vi "op_biti_v5.vi"() -> ()   [LabVIEW 2009]
panel:
  out "Boolean 2":bool=TRUE
  in  "Boolean":bool=TRUE
  out "Array 2":bool[](array[boolean])=[FALSE, FALSE, FALSE, FALSE, FALSE, FALSE, FALSE, TRUE]
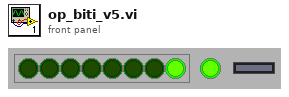
[diagram p1: front panel]
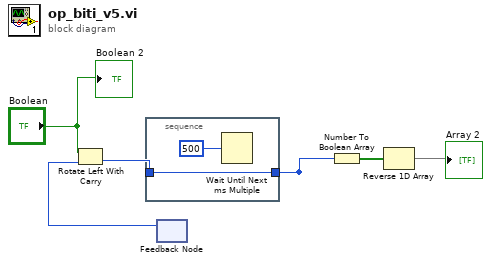
[diagram p0: block diagram]
diagram:
  n1 = feedback #1() -> (w3:u8)  [unwired: 1 in]
  n2 = Rotate Left With Carry(2:w3, 3:"Boolean") -> (0:w4:u8)  [unwired: 1 out]
  n3 = stacked-sequence {
    tunnel: w4 -> [w8]
    tunnel: [w8] -> w2
    frame #0 {
      n4 = Wait Until Next ms Multiple(millisecond multiple=500) -> ()  [unwired: 1 out]
    }
  }
  n5 = Number To Boolean Array(number=w2) -> (Boolean array=w6:bool[])
  n6 = Reverse 1D Array(array=w6) -> (reversed array=→"Array 2":bool[])
  "Boolean 2" <- "Boolean"
